vi "Insert-action-in-sequence.vi"(5 "Sequence index in":i32, 7 "Motor index":i32, 8 "error in (no error)":errorcluster, 10 "Action":refnum<class "Action.lvclass">, 11 "Available motors in":refnum<class "Motor-assembly.lvclass">) -> (0 "error out":errorcluster, 3 "Available motors out":refnum<class "Motor-assembly.lvclass">, 4 "Sequence index":i32)   [LabVIEW 2013, in "PowderDeposition.lvlib" / "Motor-assembly.lvclass"]
uses:
  Motor-assembly.lvclass
  Action/Action.lvclass
  Motor-assembly.lvclass/Motor-assembly.ctl
  Motor/Motor.lvclass
  Sequence/Action-sequence.lvclass
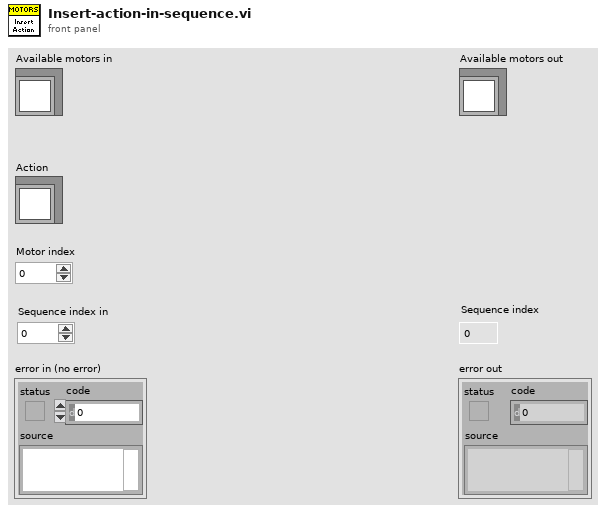
[diagram p1: front panel]
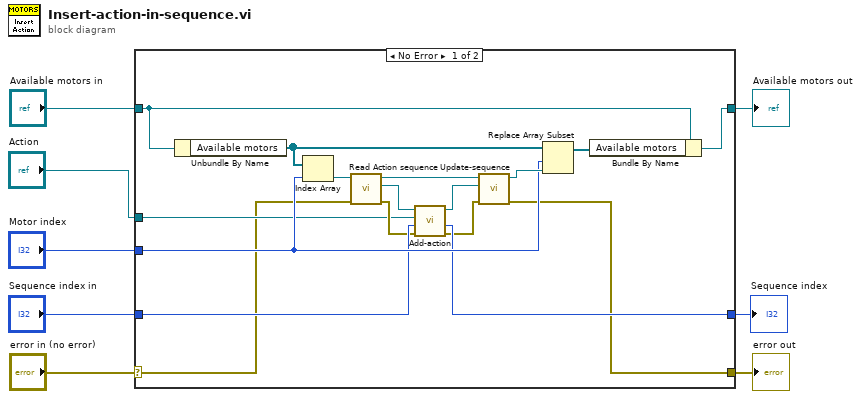
[diagram p0: block diagram]
diagram:
  n1 = case shown="No Error" "error in (no error)" {
    selector: "error in (no error)" -> [w10 w28]
    tunnel: [w9 w28] -> w7
    tunnel: [w18 w27] -> w5
    tunnel: "Available motors in" -> [w19 w27]
    tunnel: "Motor index" -> [w17 _]
    tunnel: "Sequence index in" -> [w15 w26]
    tunnel: [w14 w26] -> w2
    tunnel: "Action" -> [w12 _]
    frame No Error {
      n2 = Unbundle By Name(w19) -> ("Available motors"=w16:refnum<class "Motor.lvclass">[])
      n3 = Index Array(array=w16, index=w17) -> (element=w21:refnum<class "Motor.lvclass">)
      n4 = call-dynamic "Read Action sequence.vi"("error in (no error)"=w10, "Motor in"=w21) -> ("error out"=w13:errorcluster, "Sequence.lvclass"=w22:refnum<class "Action-sequence.lvclass">, "Motor out"=w24:refnum<class "Motor.lvclass">)  [unwired: 7 in]
      n5 = call "Add-action.vi"("error in (no error)"=w13, "Position in"=w15, "Action"=w12, "Sequence in"=w22) -> ("error out"=w11:errorcluster, "Position"=w14:i32, "Sequence out"=w23:refnum<class "Action-sequence.lvclass">)  [unwired: 5 in]
      n6 = call-dynamic "Update-sequence.vi"("error in (no error)"=w11, "Sequence"=w23, "Motor in"=w24) -> ("error out"=w9:errorcluster, "Motor out"=w25:refnum<class "Motor.lvclass">)  [unwired: 7 in]
      n7 = Replace Array Subset(array=w16, new element=w25, index=w17) -> (w20:refnum<class "Motor.lvclass">[])
      n8 = Bundle By Name(cluster=w19, "Available motors"=w20) -> (w18:refnum<class "Motor-assembly.lvclass">)
    }
    frame Error {
    }
  }
  "error out" <- w7
  "Available motors out" <- w5
  "Sequence index" <- w2
